vi "bruit gaussien.vi"() -> ()   [LabVIEW 2026]
uses:
  C:/Users/laserfab/Desktop/T-Cube TPZ001-LV2026Q1/Thorlabs.MotionControl.Controls.dll
  Thorlabs.MotionControl.Controls.dll
  C:/Users/laserfab/Desktop/T-Cube TPZ001-LV2026Q1/Thorlabs.MotionControl.TCube.PiezoCLI.dll
  Thorlabs.MotionControl.TCube.PiezoCLI.dll
  <vilib>/ptbypt/NI_PtbyPt.lvlib
panel:
  in  "stop":bool
  out "Graphe déroulant 2":dbl(graph)
  out "Graphe déroulant":dbl(graph)
  in  "TCubePiezoControl":refnum<k24>(container)
  in  "SerialNumber":string="81844665"
  out "CreateDevice":bool=TRUE
  out "GetOutputVoltage":dbl=0.00686666463209937
  out "CloseDevice":bool=TRUE
  in  "TCubePiezoControl 2":refnum<k24>(container)
  out "CreateDevice 2":bool=TRUE
  out "GetOutputVoltage 2":dbl=0.00686666463209937
  in  "SerialNumber 2":string="81844656"
  out "CloseDevice 2":bool=TRUE
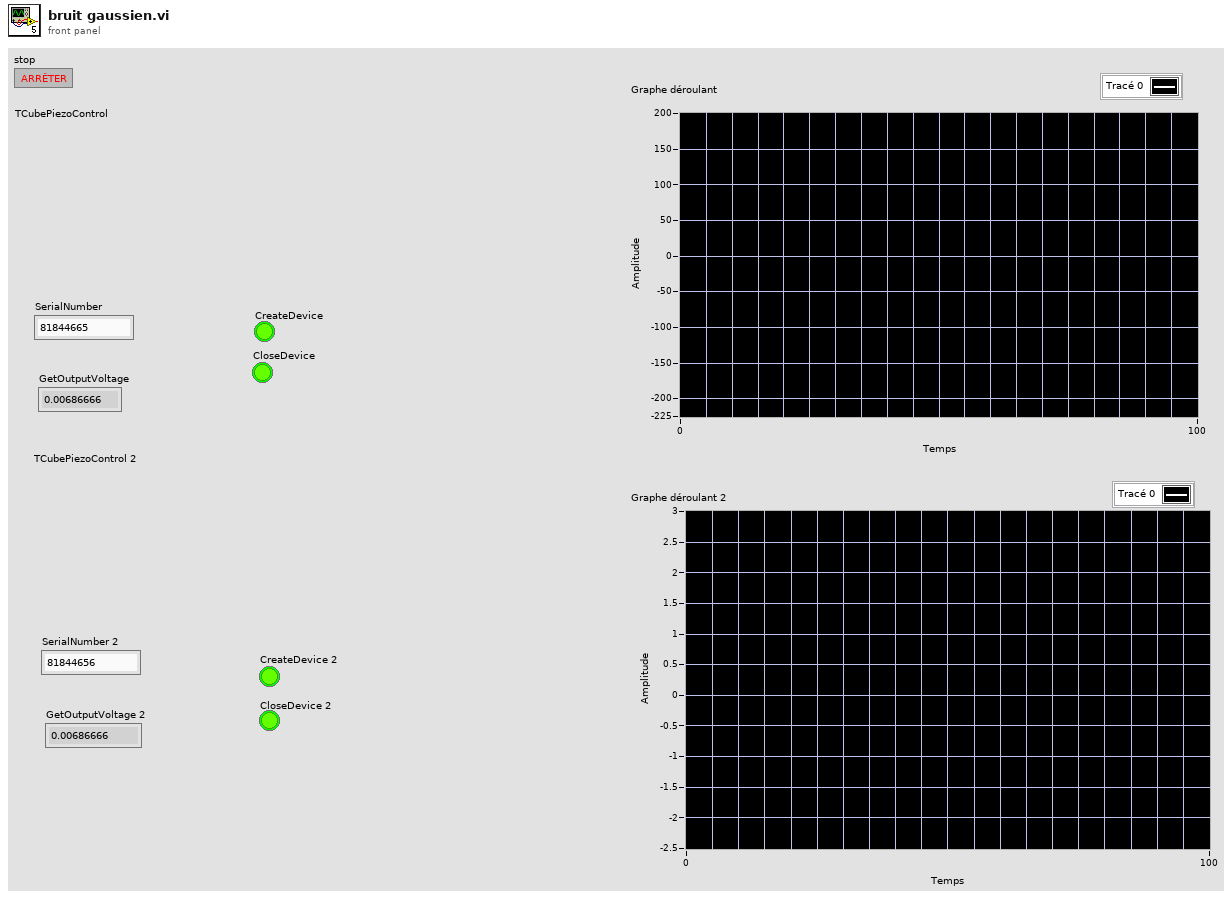
[diagram p1: front panel]
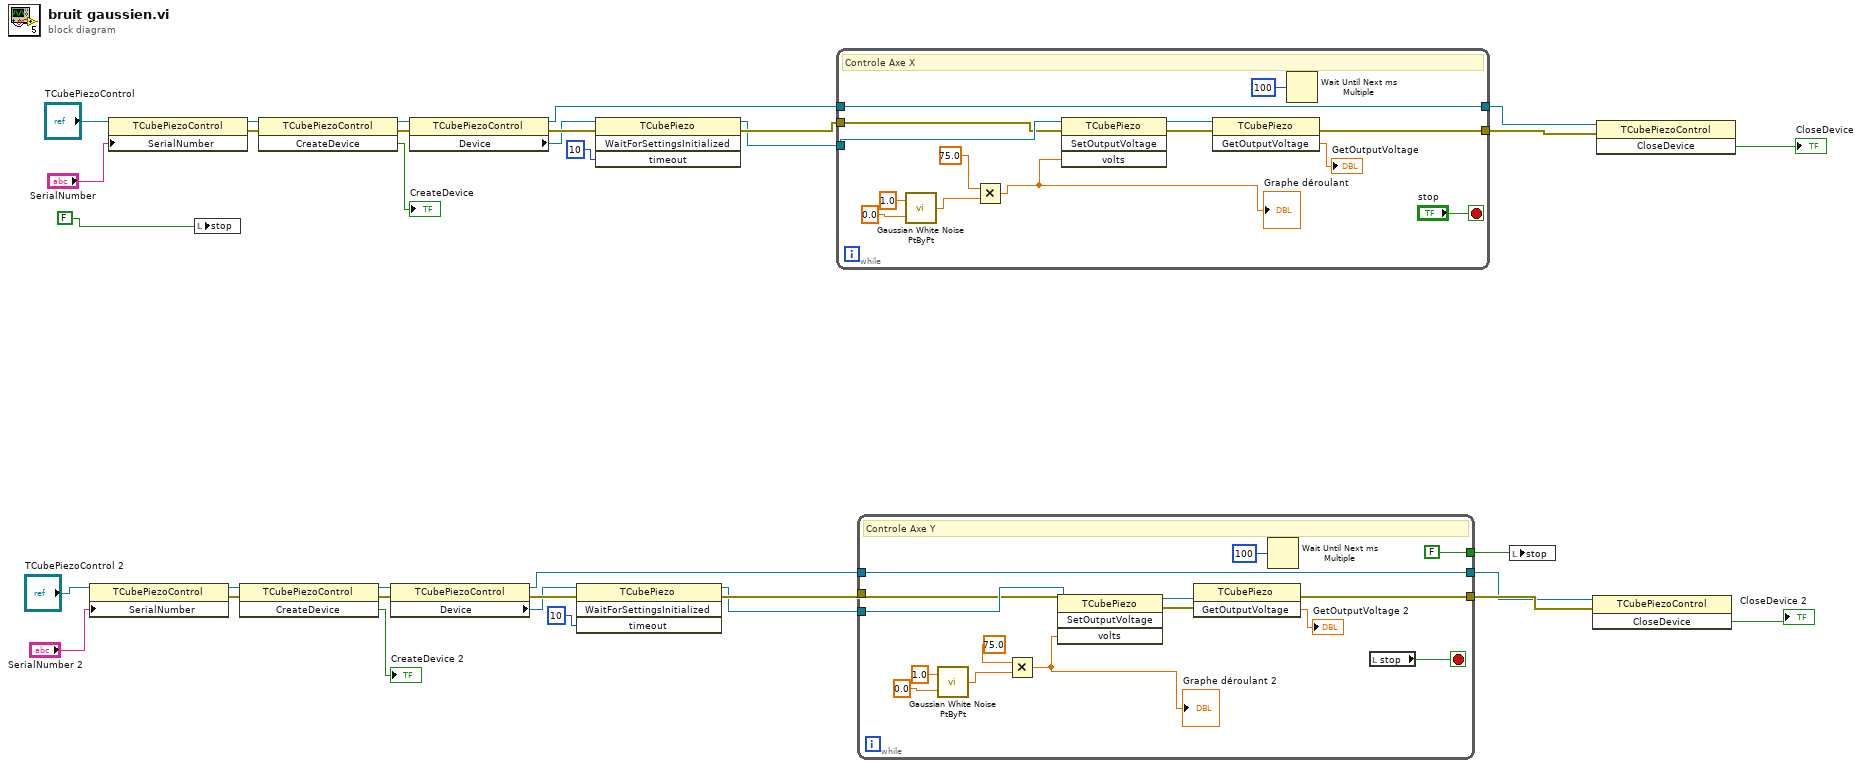
[diagram p0: block diagram]
diagram:
  n1 = property on="Nœud de propriété" class="TCubePiezoControl"(reference="TCubePiezoControl 2", "SerialNumber"="SerialNumber 2") -> (reference out=w4:refnum<k24>, error out=w5:errorcluster)  [unwired: 1 in]
  n2 = property on="Nœud de propriété" class="TCubePiezoControl"(reference="TCubePiezoControl", "SerialNumber"="SerialNumber") -> (reference out=w22:refnum<k24>, error out=w23:errorcluster)  [unwired: 1 in]
  n3 = local write "stop"(FALSE ("stop")) -> ()
  n4 = invoke on="Nœud de méthode" class="TCubePiezoControl" method="CreateDevice"(reference=w4, error in=w5) -> (reference out=w7:refnum<k24>, error out=w6:errorcluster, "CreateDevice"=→"CreateDevice 2":bool)  [unwired: 1 in]
  n5 = invoke on="Nœud de méthode" class="TCubePiezoControl" method="CreateDevice"(reference=w22, error in=w23) -> (reference out=w25:refnum<k24>, error out=w24:errorcluster, "CreateDevice"=→"CreateDevice":bool)  [unwired: 1 in]
  n6 = property on="Nœud de propriété" class="TCubePiezoControl"(reference=w7, error in=w6) -> (reference out=w9:refnum<k24>, error out=w16:errorcluster, "Device"=w14:refnum<k24>)
  n7 = property on="Nœud de propriété" class="TCubePiezoControl"(reference=w25, error in=w24) -> (reference out=w27:refnum<k24>, error out=w31:errorcluster, "Device"=w30:refnum<k24>)
  n8 = invoke on="Nœud de méthode" class="TCubePiezo" method="WaitForSettingsInitialized"(reference=w14, error in=w16, "timeout"=10) -> (reference out=w17:refnum<k24>, error out=w18:errorcluster)  [unwired: 1 in, 2 out]
  n9 = invoke on="Nœud de méthode" class="TCubePiezo" method="WaitForSettingsInitialized"(reference=w30, error in=w31, "timeout"=10) -> (reference out=w33:refnum<k24>, error out=w34:errorcluster)  [unwired: 1 in, 2 out]
  n10 = while {
    tunnel: w27 -> [w48]
    tunnel: [w48] -> w28
    tunnel: [w47] -> w29
    tunnel: w33 -> [w45]
    tunnel: w34 -> [w44]
    stop <- "stop" stop-if-true
    # "Controle Axe X"
    n11 = call <vilib>:"Gaussian White Noise PtByPt.vi"("seed"=0.0, "standard deviation"=1.0) -> ("Gaussian white noise"=w38:dbl)  [unwired: 1 in]
    n12 = Multiply(x=75.0, y=w38) -> (x*y=w36:dbl)
    "Graphe déroulant" <- w36
    n13 = invoke on="Nœud de méthode" class="TCubePiezo" method="SetOutputVoltage"(reference=w45, error in=w44, "volts"=w36) -> (reference out=w43:refnum<k24>, error out=w42:errorcluster)  [unwired: 1 in, 2 out]
    n14 = invoke on="Nœud de méthode" class="TCubePiezo" method="GetOutputVoltage"(reference=w43, error in=w42) -> (error out=w47:errorcluster, "GetOutputVoltage"=→"GetOutputVoltage":dbl)  [unwired: 1 in, 1 out]
    n15 = Wait Until Next ms Multiple(millisecond multiple=u32 100 ("n millisecondes")) -> ()  [unwired: 1 out]
  }
  n16 = while {
    tunnel: w9 -> [w63]
    tunnel: [w63] -> w10
    tunnel: [w62] -> w11
    tunnel: w17 -> [w60]
    tunnel: w18 -> [w59]
    tunnel: [FALSE ("stop")] -> w1
    stop <- w49 stop-if-true
    # "Controle Axe Y"
    n17 = call <vilib>:"Gaussian White Noise PtByPt.vi"("seed"=0.0, "standard deviation"=1.0) -> ("Gaussian white noise"=w53:dbl)  [unwired: 1 in]
    n18 = Multiply(x=75.0, y=w53) -> (x*y=w50:dbl)
    "Graphe déroulant 2" <- w50
    n19 = invoke on="Nœud de méthode" class="TCubePiezo" method="SetOutputVoltage"(reference=w60, error in=w59, "volts"=w50) -> (reference out=w58:refnum<k24>, error out=w57:errorcluster)  [unwired: 1 in, 2 out]
    n20 = invoke on="Nœud de méthode" class="TCubePiezo" method="GetOutputVoltage"(reference=w58, error in=w57) -> (error out=w62:errorcluster, "GetOutputVoltage"=→"GetOutputVoltage 2":dbl)  [unwired: 1 in, 1 out]
    n21 = Wait Until Next ms Multiple(millisecond multiple=u32 100 ("n millisecondes")) -> ()  [unwired: 1 out]
    n22 = local read "stop"() -> (w49:bool)
  }
  n23 = local write "stop"(w1) -> ()
  n24 = invoke on="Nœud de méthode" class="TCubePiezoControl" method="CloseDevice"(reference=w10, error in=w11) -> ("CloseDevice"=→"CloseDevice 2":bool)  [unwired: 1 in, 2 out]
  n25 = invoke on="Nœud de méthode" class="TCubePiezoControl" method="CloseDevice"(reference=w28, error in=w29) -> ("CloseDevice"=→"CloseDevice":bool)  [unwired: 1 in, 2 out]
